vi "gyro_data.vi"() -> ()   [LabVIEW 2014]
uses:
  <vilib>/Platform/TimedLoop/XDataNode/timing_clust.ctl
  <vilib>/Platform/TimedLoop/XDataNode/nitl_modes.ctl
  <vilib>/Platform/TimedLoop/XDataNode/wakeup.ctl
  <vilib>/Analysis/3filter.llb/Filter Passband Type.ctl
  <vilib>/myRIO/Instrument Drivers/Onboard IO/AI/vis/Read.vi
  <vilib>/myRIO/Instrument Drivers/Onboard IO/AI/vis/Smart Open.vi
  <vilib>/Utility/error.llb/Error Cluster From Error Code.vi
  <vilib>/myRIO/Common/Instrument Driver Framework/myRIO v1.0/AI/vis/myRIO v1.0 Read AI.vi
  <vilib>/platform/TimedLoop/XDataNode/XDataNode.xnode
  <vilib>/Platform/TimedLoop/XDataNode/XDNodeRunTimeDep.lvlib
  <vilib>/ptbypt/NI_PtbyPt.lvlib
  <vilib>/Analysis/NI_AALBase.lvlib
panel:
  out "Angluar Rate":dbl
  out "文件路径":path
  out "Angle_org":dbl(graph)
  in  "initialize_org":bool
  in  "initialize_Butterworth":bool
  out "Angle_Butterworth":dbl(graph)
  out "Angluar Rate_Butterworth":dbl(graph)
  out "Angle_average":dbl(graph)
  in  "initialize_average":bool
  out "Angluar Rate_average":dbl(graph)
  out "Angluar Rate":dbl(graph)
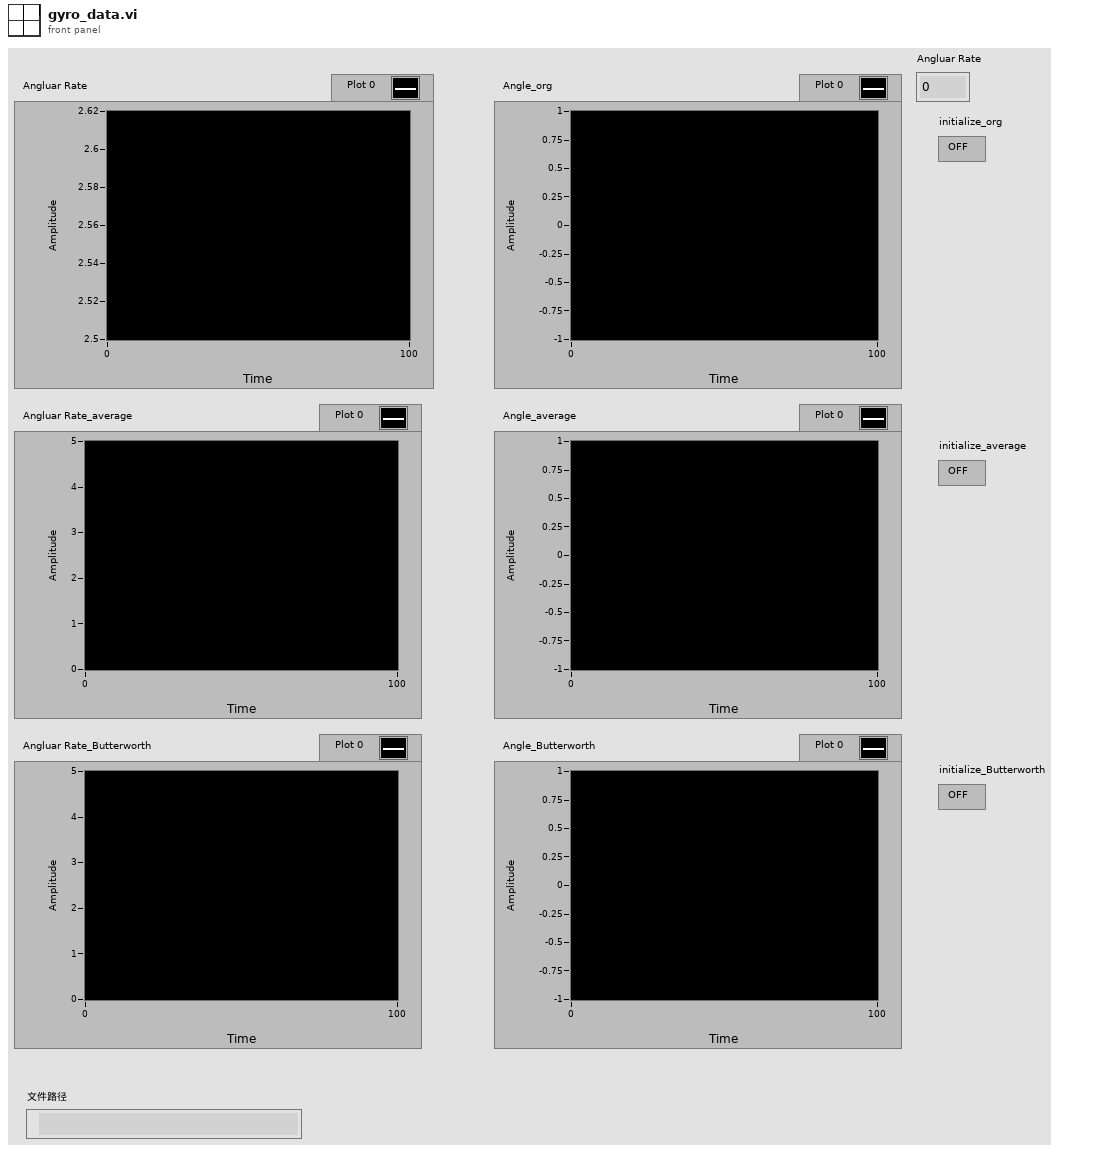
[diagram p1: front panel]
types:
  T1 = enum16{"open", "replace", "create", "open or create", "replace or create", "replace or create with confirmation"}
  T2 = typedef "XDNodeRunTimeDep.lvlib/timing_clust.ctl" = cluster{"Expected End [f-1]":u64, "Actual End [f-1]":u64, "Finished Late? [f-1]":bool, "Expected End [i-1]":u64, "Actual End [i-1]":u64, "Finished Late? [i-1]":bool, "Expected Start [i]":u64, "Actual Start [i]":u64, "Expected Start [f]":u64, "Actual Start [f]":u64, "Source Name":string, "Structure Name":string, "Period":i64, "Deadline":i64, "Offset":i64, "Start":i64, "Priority":i32, "Timeout":i32, "Mode":T3, "Wakeup Reason":T4, "Error":errorcluster, "Source Type":string, "Secondary Source Type":string, "Global End Time":u64, "Global Start Time":u64, "Frame Duration":u64, "Iteration Duration":u64, "Assigned CPU":i32, "I/O Scan Engine Mode":u32}
  T3 = typedef "XDNodeRunTimeDep.lvlib/nitl_modes.ctl" = enum32{"No Change", "Process missed periods, maintain original phase", "Discard missed periods, maintain original phase", "Process missed periods, ignore original phase", "Discard missed periods, ignore original phase"}
  T4 = typedef "XDNodeRunTimeDep.lvlib/wakeup.ctl" = enum32{"Normal", "Aborted", "Asynchronous wakeup", "Timing source error", "Timed loop error", "Timeout"}
  T5 = typedef "NI_AALBase.lvlib/Filter Passband Type.ctl" = enum32{"Lowpass", "Highpass", "Bandpass", "Bandstop"}
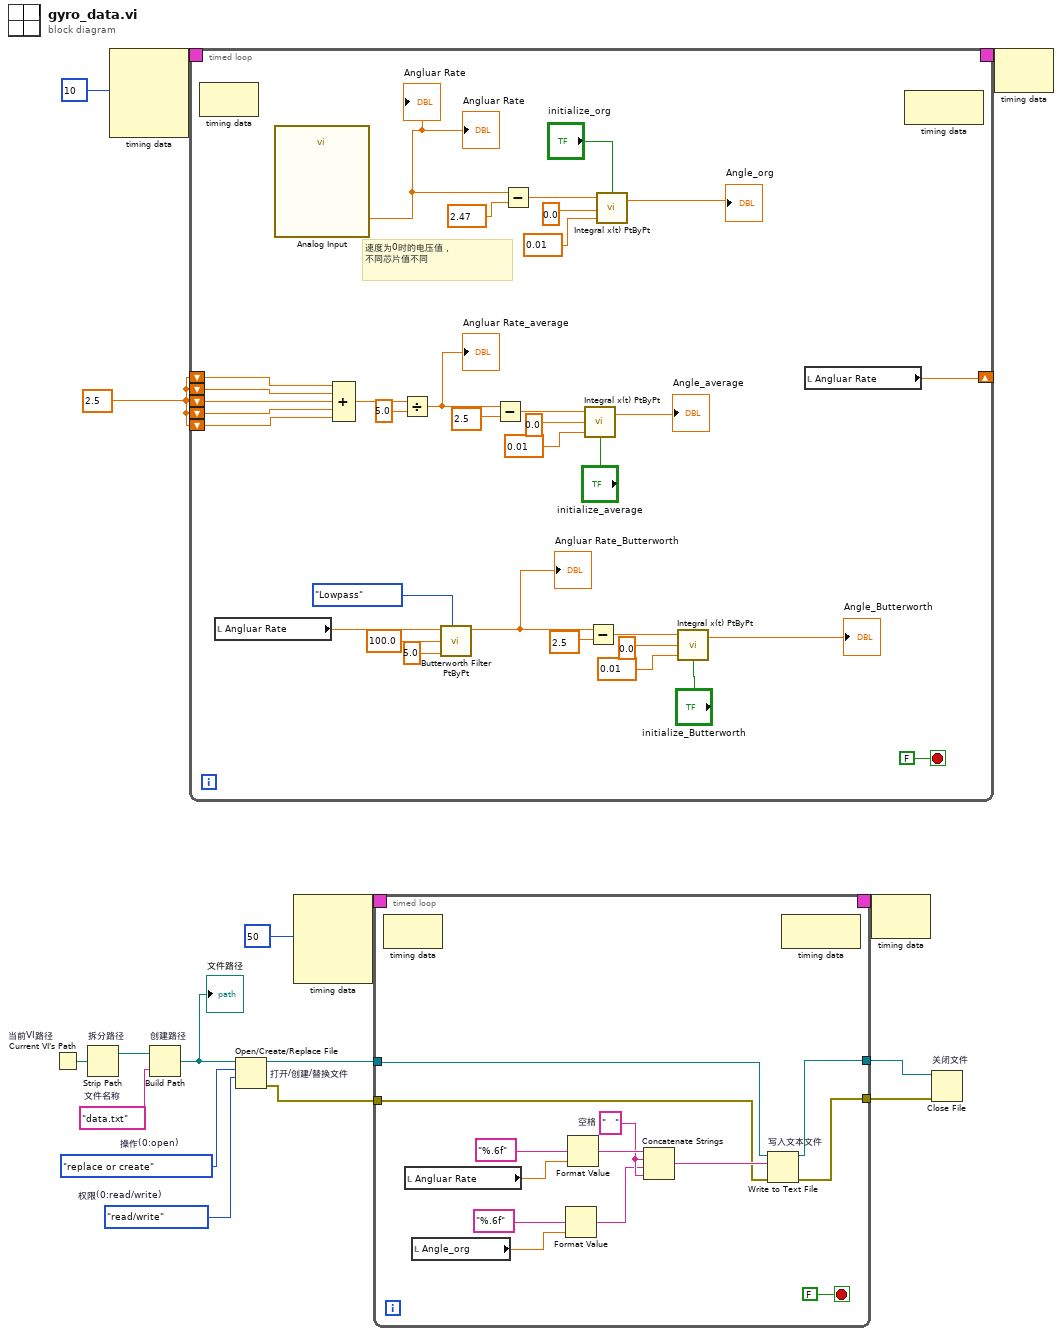
[diagram p0: block diagram]
diagram:
  w11 = "data.txt"  # 文件名称
  w12 = enum16{"read/write", "read-only", "write-only"}."read/write"  # 权限(0:read/write)
  w13 = T1."replace or create"  # 操作(0:open)
  w17 = 2.5
  n1 = Current VI's Path "当前VI路径"() -> (path=w10:path)
  n2 = Strip Path "拆分路径"(path=w10) -> (stripped path=w9:path)  [unwired: 1 out]
  n3 = node-c288(i64 10 ("Period")) -> (w16:T2)  [unwired: 3 in]
  n4 = Build Path "创建路径"(base path=w9, name or relative path=w11) -> (appended path=w8:path)
  "文件路径" <- w8
  n5 = timed-loop {
    shift-right: [w21] -> _
    shift-left: w17 -> [w51]
    shift-left: w17 -> [w50]
    shift-left: w17 -> [w49]
    shift-left: w17 -> [w48]
    shift-left: w17 -> [w47]
    timing: w16 -> [_]
    timing-out: [_] -> w15
    stop <- FALSE stop-if-true
    # "速度为0时的电压值，\n不同芯片值不同"
    n6 = node-c288() -> ()  [unwired: 1 in, 1 out]
    n7 = local read "Angluar Rate"() -> (w33:dbl)
    n8 = call "Analog Input"() -> ("B/AI0 (Pin 3)"=w20:dbl)  [unwired: 26 in, 1 out]
    "Angluar Rate" <- w20
    "Angluar Rate" <- w20
    n9 = Compound Arithmetic op=ADD(w51, w50, w49, w48, w47) -> (w46:dbl)
    n10 = Divide(x=w46, y=5.0) -> (x/y=w34:dbl)
    "Angluar Rate_average" <- w34
    n11 = call <vilib>:"Butterworth Filter PtByPt.vi"("filter type"=Filter_Passband_Type."Lowpass", "low cutoff freq: fl"=5.0, "sampling freq: fs"=100.0, "x"=w33) -> ("Filtered x"=w27:dbl)  [unwired: 5 in, 1 out]
    "Angluar Rate_Butterworth" <- w27
    n12 = Subtract(x=w34, y=2.5) -> (x-y=w42:dbl)
    n13 = Subtract(x=w20, y=2.47) -> (x-y=w25:dbl)
    n14 = call <vilib>:"Integral x(t) PtByPt.vi"("initialize"="initialize_average", "dt"=0.01, "initial condition"=0.0, "x"=w42) -> ("integral x(t)"=→"Angle_average":dbl)  [unwired: 1 out]
    n15 = Subtract(x=w27, y=2.5) -> (x-y=w28:dbl)
    n16 = call <vilib>:"Integral x(t) PtByPt.vi"("initialize"="initialize_org", "dt"=0.01, "initial condition"=0.0, "x"=w25) -> ("integral x(t)"=→"Angle_org":dbl)  [unwired: 1 out]
    n17 = call <vilib>:"Integral x(t) PtByPt.vi"("initialize"="initialize_Butterworth", "dt"=0.01, "initial condition"=0.0, "x"=w28) -> ("integral x(t)"=→"Angle_Butterworth":dbl)  [unwired: 1 out]
    n18 = local read "Angluar Rate"() -> (w21:dbl)
    n19 = node-c288() -> ()  [unwired: 1 in, 1 out]
  }
  n20 = Open/Create/Replace File "打开/创建/替换文件"(file path (use dialog)=w8, operation (0:open)=w13, access (0:read/write)=w12) -> (refnum out=w3:refnum<file>, error out=w2:errorcluster)  [unwired: 1 in, 3 out]
  n21 = node-c288(50 ("Priority")) -> (w7:T2)  [unwired: 3 in]
  n22 = timed-loop {
    timing: w7 -> [_]
    timing-out: [_] -> w6
    tunnel: w3 -> [w63]
    tunnel: w2 -> [w62]
    tunnel: [w60] -> w5
    tunnel: [w59] -> w4
    stop <- FALSE stop-if-true
    w55 = "   "  # 空格
    n23 = node-c288() -> ()  [unwired: 1 in, 1 out]
    n24 = local read "Angluar Rate"() -> (w58:dbl)
    n25 = local read "Angle_org"() -> (w57:dbl)
    n26 = Format Value(format string="%.6f", value (0)=w57) -> (output string=w54:string)  [unwired: 1 in]
    n27 = Format Value(format string="%.6f", value (0)=w58) -> (output string=w65:string)  [unwired: 1 in]
    n28 = Concatenate Strings(w65, w55, w54, w55) -> (w64:string)
    n29 = Write to Text File "写入文本文件"(file (use dialog)=w63, text=w64, error in=w62) -> (refnum out=w60:refnum<file>, error out=w59:errorcluster)  [unwired: 2 out]
    n30 = node-c288() -> ()  [unwired: 1 in, 1 out]
  }
  n31 = node-c288(w6) -> ()  [unwired: 1 out]
  n32 = Close File "关闭文件"(refnum=w5, error in=w4) -> ()  [unwired: 2 out]
  n33 = node-c288(w15) -> ()  [unwired: 1 out]
